vi "PyArgsToList.vi"(0 "Arg1":string, 1 "Arg2":string, 2 "Arg3":string, 3 "Arg4":string, 4 "Arg5":string) -> (5 "PythonList":string)   [LabVIEW 2014]
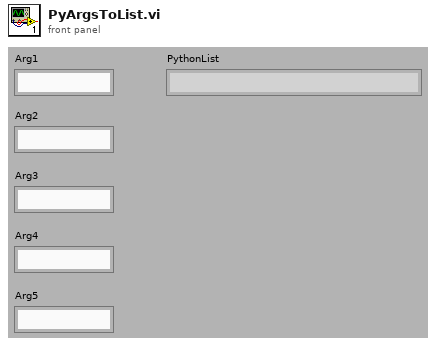
[diagram p1: front panel]
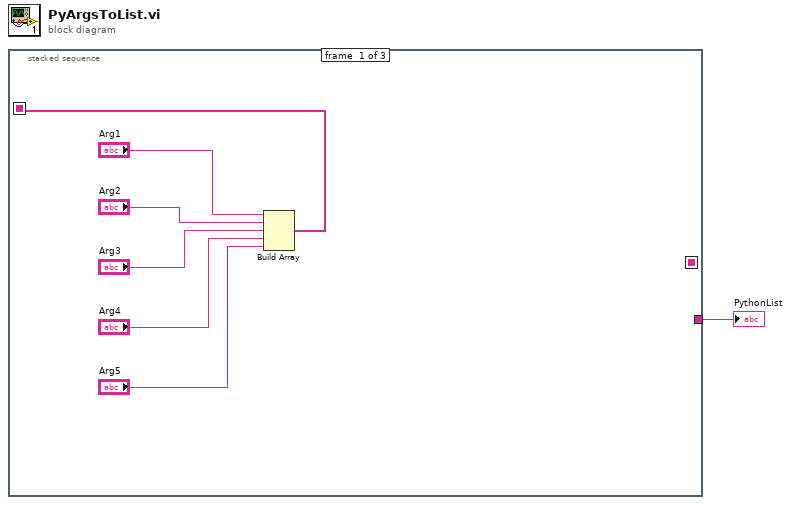
[diagram p0: block diagram]
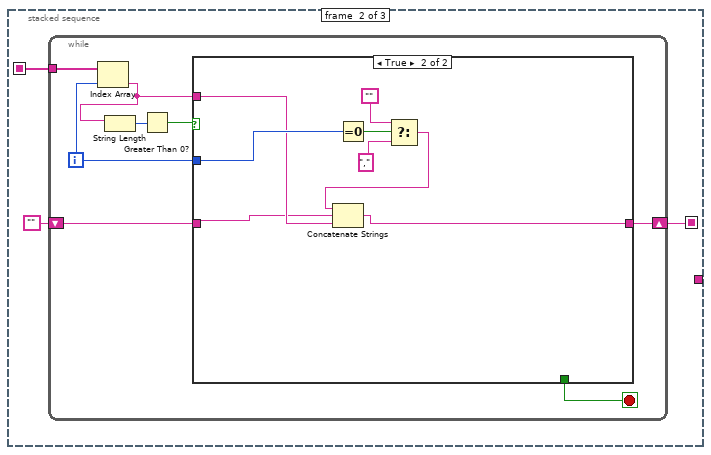
[diagram p2: hidden frame]
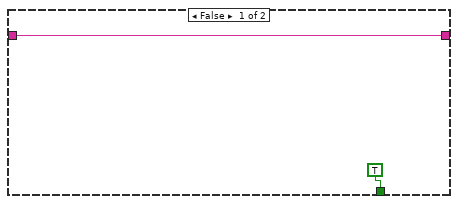
[diagram p3: hidden frame]
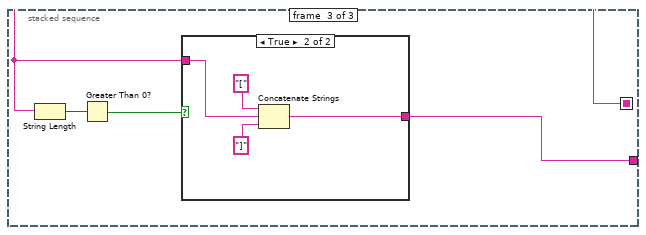
[diagram p4: hidden frame]
diagram:
  n1 = stacked-sequence {
    seq-local: [w2 _ _] -> [_ w10 _]
    seq-local: [_ w8 _] -> [_ _ w30]
    tunnel: [_ _ w29] -> w1
    frame #0 {
      n2 = Build Array("Arg1", "Arg2", "Arg3", "Arg4", "Arg5") -> (w2:string[])
    }
    frame #1 {
      n3 = while {
        tunnel: w10 -> [w18]
        shift-right: [w14] -> w8
        shift-left: "" -> [w15]
        i -> [w12]
        stop <- w11 stop-if-true
        n4 = Index Array(array=w18, index=w12) -> (element=w13:string)
        n5 = String Length(string=w13) -> (length=w17:i32)
        n6 = Greater Than 0?(x=w17) -> (x > 0?=w16:bool)
        n7 = case shown="True" w16 {
          tunnel: w15 -> [w20 w21]
          tunnel: [w20 w28] -> w14
          tunnel: w13 -> [_ w22]
          tunnel: w12 -> [_ w27]
          tunnel: [TRUE _] -> w11
          frame False {
          }
          frame True {
            n8 = Equal To 0?(x=w27) -> (x = 0?=w26:bool)
            n9 = Select(t="", s=w26, f=",") -> (s? t:f=w23:string)
            n10 = Concatenate Strings(w23, w21, w22) -> (w28:string)
          }
        }
      }
    }
    frame #2 {
      n11 = String Length(string=w30) -> (length=w32:i32)
      n12 = Greater Than 0?(x=w32) -> (x > 0?=w31:bool)
      n13 = case shown="True" w31 {
        tunnel: w30 -> [w33 w35]
        tunnel: [w33 w34] -> w29
        frame False {
        }
        frame True {
          n14 = Concatenate Strings("[", w35, "]") -> (w34:string)
        }
      }
    }
  }
  "PythonList" <- w1
